vi "ModbusRxHealthAndStatusUpdateLoop.vi"(11 "ModbusPortSettings":T1={"TxPort"="ModbusPort1Tx", "TxDataFIFO"="ModbusPort1TxFIFO", "TxInternalDataFIFO"="ModbusPort1TxInternalFIFO", "TxHealthAndStatusFIFO"="ModbusPort1TxHealthAndStatusFIFO", "RxPort"="ModbusPort1Rx", "RxDataFIFO"="ModbusPort1RxFIFO", "RxHealthAndStatusFIFO"="ModbusPort1RxHealthAndStatusFIFO", "BaseHealthAndStatusAddress"=0, "WaitForRxFrameRegister"="ModbusPort1WaitForRxControl", "IRQAddress"=0, "TriggerIRQRegister"="ModbusPort1IRQControl", "InternalHealthAndStatusFIFO"="InternalHealthAndStatusFIFO", "SoftwareControlledTrigger"="ModbusSoftwareControlledTrigger", "TimestampRegister"="TimestampRegister", "TxTimestampFIFO"="ModbusPort1TimestampFIFO"}) -> ()   [LabVIEW 2016, in "FPGAModbus.lvlib"]
uses:
  FPGAModbus.lvlib
  DataTypes/ModbusPortSettings.ctl
  <vilib>/rvi/Emulation/niFpgaGetClockAttributes.vi
  <vilib>/rvi/Emulation/niFpgaSctlEmulationGetInTimedLoop.vi
  <vilib>/rvi/Emulation/niFpgaEmulationReportErrorSimple.vi
  <vilib>/rvi/DataTransferAndStorage/Container/Common/niFpgaContainerExecOnDevCompGetState.vi
  <vilib>/rvi/Emulation/niFpgaEmulationIsFPGAContextNoSignature.vi
  <vilib>/rvi/errors/niFpgaSetErrorForExecOnDevCompSimple.vi
  <vilib>/rvi/eio/common/nirviEmuReportErrorAndStop.vi
  <vilib>/rvi/DataTransferAndStorage/Container/Common/niFpgaContainerGetUniqueNameForEmu.vi
  <vilib>/rvi/FIFO/Fifo_Resource/nirvififoEmulationSetSize.vi
  <vilib>/rvi/FIFO/Fifo_Resource/nirviFifoEmulationQueueMgr.vi
  <instcachedir>/0/nirviFifoEmulationQueueMgr_E5CAEC123FF24DC58D834DCA3CDAA9B5.lvgen/nirviFifoEmulationQueueMgr_E5CAEC123FF24DC58D834DCA3CDAA9B5_001.vi
  <vilib>/rvi/FIFO/Fifo_Resource/nirvififoEmulationDetermineInputValidOut.vi
  <vilib>/rvi/FIFO/Fifo_Resource/nirvififoEmulationCreateLock.vi
  <vilib>/rvi/Emulation/niFpgaProcessEmulError.vi
  <vilib>/rvi/FIFO/Fifo_Resource/nirvififoEmulationObtainLock.vi
  <vilib>/rvi/FIFO/Fifo_Resource/nirvififoEmulationReleaseLock.vi
  <vilib>/rvi/occurrence/nirviWaitOnOccurrenceBase.vi
  <vilib>/rvi/errors/nirviReportUnexpectedCaseInternalError.vi
  <vilib>/rvi/errors/nirviReportUnexpectedCaseInternalError (U32).vi
  <vilib>/Utility/error.llb/Clear Errors.vi
  <vilib>/rvi/interface/RandomDataEmulation/niFpgaRandomDataHandleErrors.vi
  <vilib>/rvi/Emulation/niFpgaCriticalErrorInLSC.vi
  <vilib>/rvi/DataTransferAndStorage/Container/XNode/niFpgaContainer.xnode
  <vilib>/rvi/FIFO/Fifo_Resource/niFpgaFifoEmulationRefIn.vi
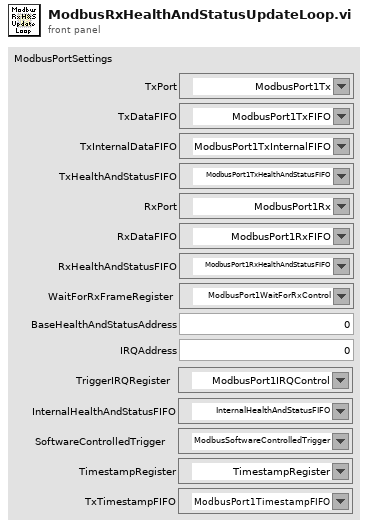
[diagram p1: front panel]
types:
  T1 = typedef "FPGAModbus.lvlib/ModbusPortSettings.ctl" = cluster{"TxPort":refnum<k21>, "TxDataFIFO":refnum<k21>, "TxInternalDataFIFO":refnum<k21>, "TxHealthAndStatusFIFO":refnum<k21>, "RxPort":refnum<k21>, "RxDataFIFO":refnum<k21>, "RxHealthAndStatusFIFO":refnum<k21>, "BaseHealthAndStatusAddress":u32, "WaitForRxFrameRegister":refnum<k21>, "IRQAddress":u8, "TriggerIRQRegister":refnum<k21>, "InternalHealthAndStatusFIFO":refnum<k21>, "SoftwareControlledTrigger":refnum<k21>, "TimestampRegister":refnum<k21>, "TxTimestampFIFO":refnum<k21>}
  T2 = cluster{"Address":u32, "Telemetry Update Mode":enum8{"NOP", "Set", "Add", "Subtract", "Or"}, "Data":u32}
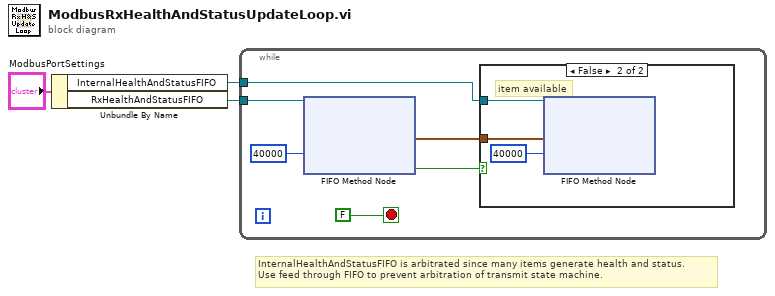
[diagram p0: block diagram]
diagram:
  # "InternalHealthAndStatusFIFO is arbitrated since many items generate health and status.\nUse feed through FIFO to prevent arbitration of transmit state machine."
  n1 = Unbundle By Name("ModbusPortSettings") -> ("InternalHealthAndStatusFIFO"=w1:refnum<k21>, "RxHealthAndStatusFIFO"=w2:refnum<k21>)
  n2 = while {
    tunnel: w2 -> [w8]
    tunnel: w1 -> [w5]
    stop <- FALSE stop-if-true
    n3 = xnode ("FIFO Method Node")("Timeout"=40000, "FIFO In"=w8) -> ("Element"=w9:T2, "Timed Out?"=w6:bool)  [unwired: 1 out]
    n4 = case shown="False" w6 {
      tunnel: w9 -> [_ w11]
      tunnel: w5 -> [_ w10]
      frame True {
        # "no item available"
      }
      frame False {
        # "item available"
        n5 = xnode ("FIFO Method Node")("Element"=w11, "Timeout"=40000, "FIFO In"=w10) -> ()  [unwired: 2 out]
      }
    }
  }
